vi "Display7seg_2digitos.vi"() -> ()   [LabVIEW 2020]
panel:
  out "appended array":bool[](array[boolean])
  out "Unidades 2":i32=9
  out "Decenas 2":i32=9
  in  "Decenas":i32=9
  in  "Unidades":i32=9
  in  "Numeric 3":i32
  out "Display 2":bool
  out "Display1":bool
  in  "Stop":bool
  out "c":bool
  out "d":bool
  out "e":bool
  out "g":bool
  out "f":bool
  out "b":bool
  out "a":bool
  in  "Digito":i32=8
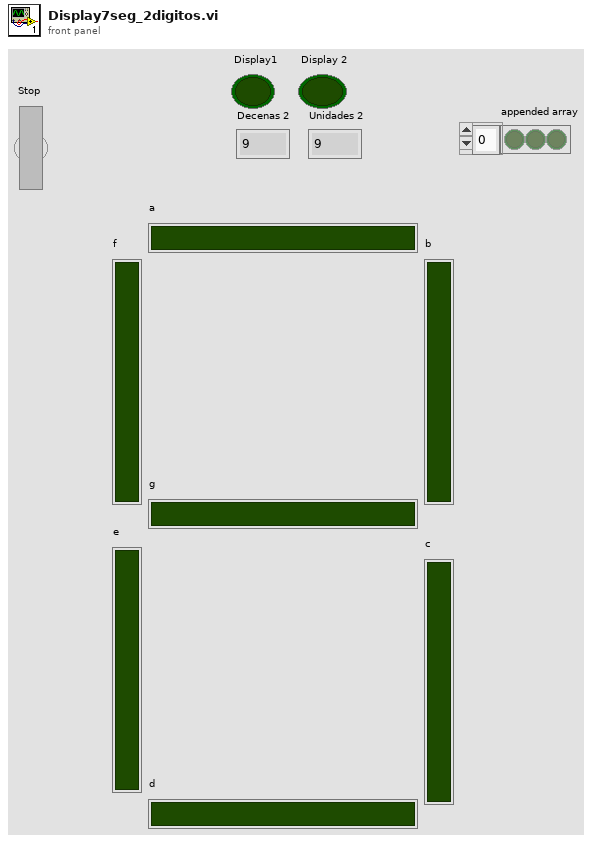
[diagram p1: front panel]
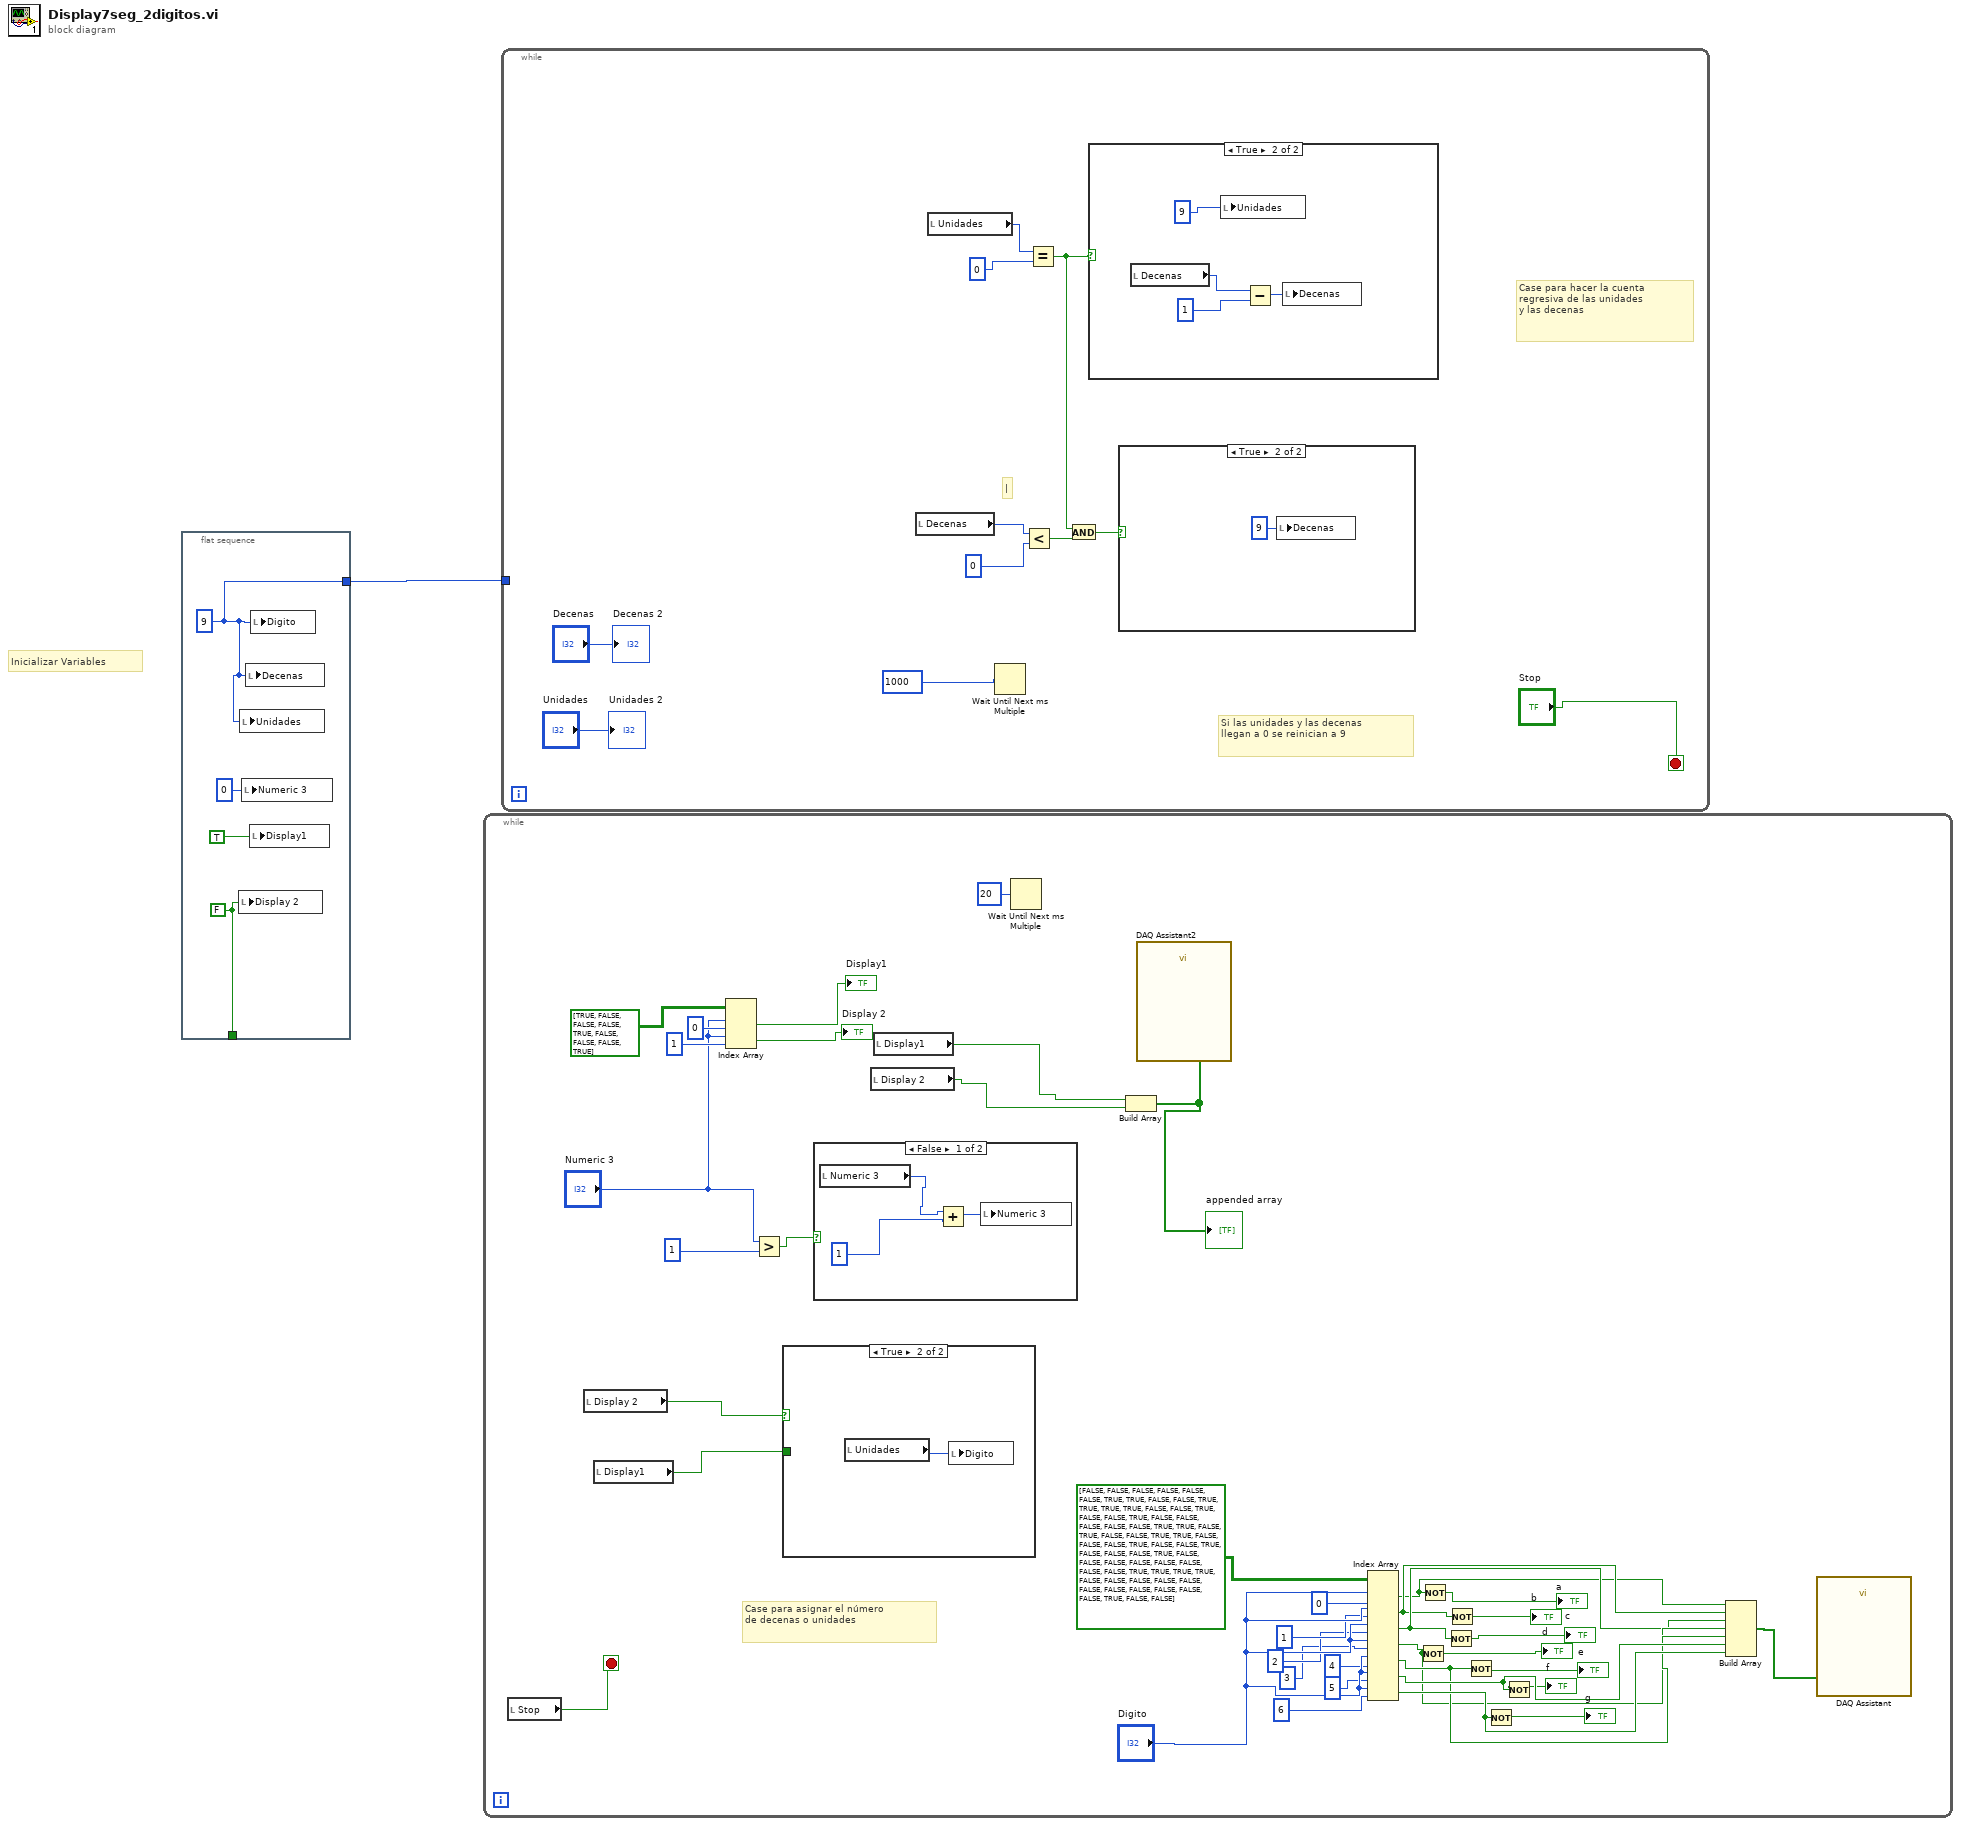
[diagram p0: block diagram]
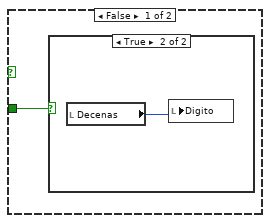
[diagram p2: hidden frame]
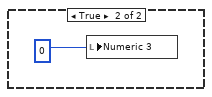
[diagram p4: hidden frame]
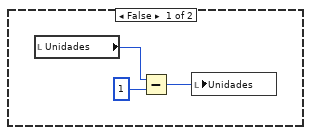
[diagram p6: hidden frame]
diagram:
  # "Inicializar Variables"
  n1 = flat-sequence {
    tunnel: [w3] -> w1
    tunnel: [w4] -> _
    frame #0 {
      w4 = FALSE
      w3 = 9 ("Numeric")
      n2 = local write "Display 2"(w4) -> ()
      n3 = local write "Unidades"(w3) -> ()
      n4 = local write "Numeric 3"(0 ("Numeric 3")) -> ()
      n5 = local write "Decenas"(w3) -> ()
      n6 = local write "Display1"(TRUE) -> ()
      n7 = local write "Digito"(w3) -> ()
    }
  }
  n8 = while {
    stop <- w44 stop-if-true
    # "Case para asignar el número\nde decenas o unidades"
    n9 = local read "Stop"() -> (w44:bool)
    n10 = local read "Display 2"() -> (w30:bool)
    n11 = local read "Display1"() -> (w31:bool)
    n12 = Index Array(array=bool[][] [[TRUE, FALSE, FALSE], [FALSE, TRUE, FALSE], [FALSE, FALSE, TRUE]], index (row) #1="Numeric 3", index (col) #1=0 ("disabled index (col)"), index (row) #2="Numeric 3", index (col) #2=1 ("index (col)")) -> (element #1=→"Display1":bool, element #2=→"Display 2":bool)
    n13 = Greater?(x="Numeric 3", y=1) -> (0:w35:bool)
    n14 = case shown="True" w30 {
      tunnel: w31 -> [w45 _]
      frame False {
        n15 = case shown="True" w45 {
          frame False {
          }
          frame True {
            n16 = local read "Decenas"() -> (w46:i32)
            n17 = local write "Digito"(w46) -> ()
          }
        }
      }
      frame True {
        n18 = local read "Unidades"() -> (w47:i32)
        n19 = local write "Digito"(w47) -> ()
      }
    }
    n20 = case shown="False" w35 {
      frame False {
        n21 = local read "Numeric 3"() -> (w48:i32)
        n22 = Add(x=w48, y=1 ("x")) -> (x+y=w50:i32)
        n23 = local write "Numeric 3"(w50) -> ()
      }
      frame True {
        n24 = local write "Numeric 3"(0) -> ()
      }
    }
    n25 = local read "Display 2"() -> (w33:bool)
    n26 = local read "Display1"() -> (w32:bool)
    n27 = Wait Until Next ms Multiple(millisecond multiple=u32 20) -> ()  [unwired: 1 out]
    n28 = Build Array(w32, w33) -> (w34:bool[])
    "appended array" <- w34
    n29 = call "DAQ Assistant2"("data"=w34) -> ()  [unwired: 17 in, 2 out]
    n30 = Index Array "Index Array"(array=bool[][] [[FALSE, FALSE, FALSE, FALSE, FALSE, FALSE, TRUE], [TRUE, FALSE, FALSE, TRUE, TRUE, TRUE, TRUE], [FALSE, FALSE, TRUE, FALSE, FALSE, TRUE, FALSE], [FALSE, FALSE, FALSE, FALSE, TRUE, TRUE, FALSE], [TRUE, FALSE, FALSE, TRUE, TRUE, FALSE, FALSE], [FALSE, TRUE, FALSE, FALSE, TRUE, FALSE, FALSE], [FALSE, TRUE, FALSE, FALSE, FALSE, FALSE, FALSE], [FALSE, FALSE, FALSE, TRUE, TRUE, TRUE, TRUE], [FALSE, FALSE, FALSE, FALSE, FALSE, FALSE, FALSE], [FALSE, FALSE, FALSE, FALSE, TRUE, FALSE, FALSE]], index (row) #1="Digito", index (col) #1=0 ("disabled index (col)"), index (row) #2="Digito", index (col) #2=1 ("disabled index (col)"), index (row) #3="Digito", index (col) #3=2 ("disabled index (col)"), index (row) #4="Digito", index (col) #4=3 ("disabled index (col)"), index (row) #5="Digito", index (col) #5=4 ("disabled index (col)"), index (row) #6="Digito", index (col) #6=5 ("disabled index (col)"), index (row) #7="Digito", index (col) #7=6 ("disabled index (col)")) -> (element #1=w22:bool, element #2=w23:bool, element #3=w24:bool, element #4=w25:bool, element #5=w26:bool, element #6=w27:bool, element #7=w28:bool)
    n31 = Not(x=w25) -> (.not. x?=→"d":bool)
    n32 = Not(x=w22) -> (.not. x?=→"a":bool)
    n33 = Not(x=w24) -> (.not. x?=→"c":bool)
    n34 = Not(x=w23) -> (.not. x?=→"b":bool)
    n35 = Not(x=w26) -> (.not. x?=→"e":bool)
    n36 = Not(x=w28) -> (.not. x?=→"g":bool)
    n37 = Not(x=w27) -> (.not. x?=→"f":bool)
    n38 = Build Array(w22, w23, w24, w25, w26, w27, w28) -> (w29:bool[])
    n39 = call "DAQ Assistant"("data"=w29) -> ()  [unwired: 17 in, 2 out]
  }
  n40 = while {
    tunnel: w1 -> [_]
    stop <- "Stop" stop-if-true
    # "|"
    # "Case para hacer la cuenta\nregresiva de las unidades \ny las decenas"
    # "Si las unidades y las decenas\nllegan a 0 se reinician a 9"
    n41 = local read "Decenas"() -> (w54:i32)
    n42 = local read "Unidades"() -> (w61:i32)
    n43 = Wait Until Next ms Multiple(millisecond multiple=u32 1000 ("milliseconds to wait")) -> ()  [unwired: 1 out]
    n44 = Less?(x=w54, y=0) -> (x < y?=w55:bool)
    n45 = Equal?(x=w61, y=0) -> (x = y?=w58:bool)
    n46 = And(x=w58, y=w55) -> (x .and. y?=w59:bool)
    n47 = case shown="True" w58 {
      frame False {
        n48 = local read "Unidades"() -> (w66:i32)
        n49 = Subtract(x=w66, y=1) -> (x-y=w64:i32)
        n50 = local write "Unidades"(w64) -> ()
      }
      frame True {
        n51 = local read "Decenas"() -> (w69:i32)
        n52 = local write "Unidades"(9) -> ()
        n53 = Subtract(x=w69, y=1) -> (x-y=w67:i32)
        n54 = local write "Decenas"(w67) -> ()
      }
    }
    n55 = case shown="True" w59 {
      frame False {
      }
      frame True {
        n56 = local write "Decenas"(9 ("Decenas")) -> ()
      }
    }
    "Decenas 2" <- "Decenas"
    "Unidades 2" <- "Unidades"
  }
